vi "SignalGenerator_4.vi"(10 "Phase":fxp<+,64,64>[](array[numeric])=[0.0, 0.0, 0.0, 0.0], 11 "reset":bool) -> (1 "Sine out":fxp<+/-,16,0>[](array[numeric]), 2 "Cosine out":fxp<+/-,16,0>[](array[numeric]))   [LabVIEW 2013]
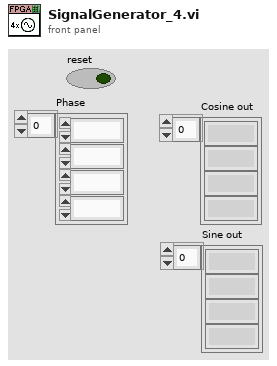
[diagram p1: front panel]
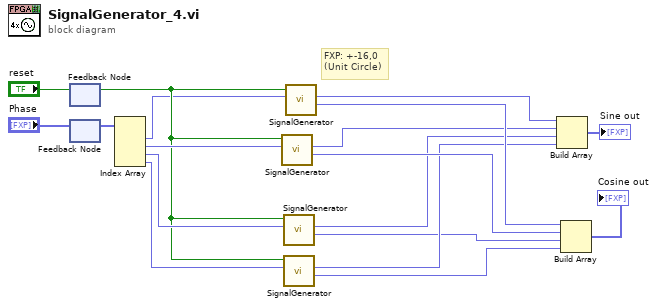
[diagram p0: block diagram]
diagram:
  # "FXP: +-16,0\n(Unit Circle)"
  n1 = feedback #1() -> (w10:bool)  [unwired: 1 in]
  n2 = feedback-in #1("reset") -> ()
  n3 = feedback #2() -> (w12:fxp<+,64,64>[])  [unwired: 1 in]
  n4 = feedback-in #2("Phase") -> ()
  n5 = Index Array(array=w12) -> (element #1=w9:fxp<+,64,64>, element #2=w16:fxp<+,64,64>, element #3=w15:fxp<+,64,64>, element #4=w14:fxp<+,64,64>)  [unwired: 4 in]
  n6 = call "SignalGenerator.vi"("phase"=w16, "Reset"=w10) -> ("Cos"=w5:fxp<+/-,16,0>, "Sin"=w6:fxp<+/-,16,0>)  [unwired: 7 in, 1 out]
  n7 = call "SignalGenerator.vi"("phase"=w15, "Reset"=w10) -> ("Cos"=w2:fxp<+/-,16,0>, "Sin"=w4:fxp<+/-,16,0>)  [unwired: 7 in, 1 out]
  n8 = call "SignalGenerator.vi"("phase"=w14, "Reset"=w10) -> ("Cos"=w1:fxp<+/-,16,0>, "Sin"=w3:fxp<+/-,16,0>)  [unwired: 7 in, 1 out]
  n9 = call "SignalGenerator.vi"("phase"=w9, "Reset"=w10) -> ("Cos"=w7:fxp<+/-,16,0>, "Sin"=w8:fxp<+/-,16,0>)  [unwired: 7 in, 1 out]
  n10 = Build Array(w8, w6, w4, w3) -> (→"Sine out":fxp<+/-,16,0>[])
  n11 = Build Array(w7, w5, w2, w1) -> (→"Cosine out":fxp<+/-,16,0>[])
